vi "Sort and Index (DBL).vi"(4 "X":dbl[](array[numeric])) -> (0 "Index":i32[](array[numeric]), 1 "Sort(X)":dbl[](array[numeric]))   [LabVIEW 2020]
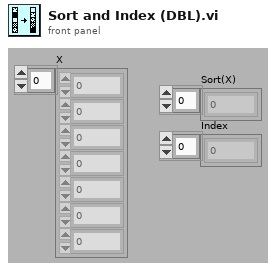
[diagram p1: front panel]
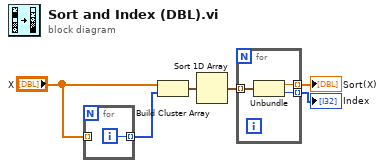
[diagram p0: block diagram]
diagram:
  n1 = for {
    tunnel: "X" -> [_] mode=indexing
    tunnel: [w7] -> w3 mode=indexing
    i -> [w7]
  }
  n2 = Build Cluster Array("X", w3) -> (w6:cluster{"value":dbl, i32}[])
  n3 = Sort 1D Array(array=w6) -> (sorted array=w5:cluster{"value":dbl, i32}[])
  n4 = for {
    tunnel: w5 -> [w10] mode=indexing
    tunnel: [w9] -> w1 mode=indexing
    tunnel: [w8] -> w2 mode=indexing
    n5 = Unbundle(w10) -> ("value"=w8:dbl, w9:i32)
  }
  "Sort(X)" <- w2
  "Index" <- w1
